vi "Set Multicolumn Listbox Column Width.vi"(5 "Number of Columns":i32, 6 "Auto Columns":bool=TRUE, 7 "Number of Rows":u32=42, 10 "error in (no error)":errorcluster, 11 "Multicolumn ListBox":refnum<vi>) -> (2 "error out":errorcluster, 3 "reference out":refnum<vi>)   [LabVIEW 2017]
uses:
  <vilib>/Utility/miscctls.llb/LVRowAndColumnTypeDef.ctl
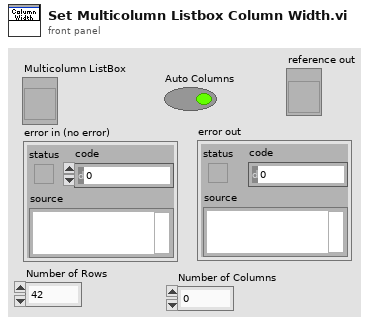
[diagram p1: front panel]
types:
  T1 = typedef "LVRowAndColumnTypeDef.ctl" = cluster{"Row":i32, "Column":i32}
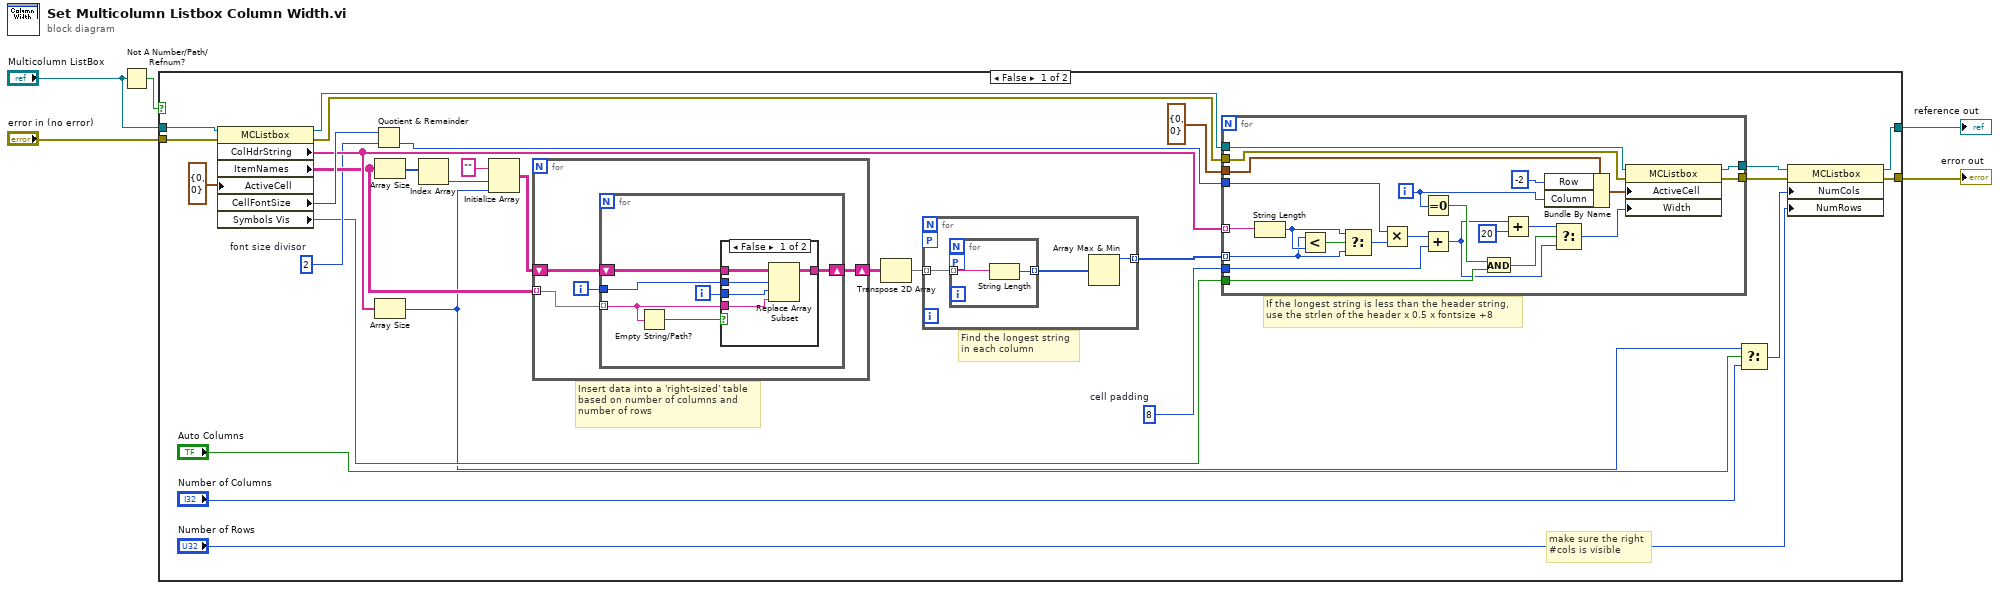
[diagram p0: block diagram]
diagram:
  n1 = Not A Number/Path/Refnum?(number/path/refnum="Multicolumn ListBox") -> (NaN/Path/Refnum?=w3:bool)
  n2 = case shown="False" w3 {
    tunnel: "Multicolumn ListBox" -> [w19 w79]
    tunnel: "error in (no error)" -> [w14 w80]
    tunnel: [w13 w80] -> w4
    tunnel: [w7 w79] -> w1
    frame False {
      w20 = u32 8  # cell padding
      w22 = u32 2  # font size divisor
      # "make sure the right\n#cols is visible"
      # "If the longest string is less than the header string,\nuse the strlen of the header x 0.5 x fontsize +8"
      # "Find the longest string\nin each column"
      # "Insert data into a 'right-sized' table\nbased on number of columns and\nnumber of rows"
      n3 = property on="Property Node" class="MCListbox"(reference=w19, error in=w14, "ActiveCell"=T1 {"Row"=0, "Column"=0} ("Active Cell:Active Cell")) -> (reference out=w15:refnum<vi>, error out=w18:errorcluster, "ColHdrString"=w25:string[], "ItemNames"=w24:string[][], "CellFontSize"=w30:u32, "Symbols Vis"=w12:bool)
      n4 = Quotient & Remainder(x=w30, y=w22) -> (floor(x/y)=w21:u32)  [unwired: 1 out]
      n5 = Array Size(array=w24) -> (size(s)=w28:i32[])
      n6 = Array Size(array=w25) -> (size(s)=w6:i32)
      n7 = Index Array(array=w28) -> (element=w29:i32)  [unwired: 1 in]
      n8 = Initialize Array("", w29, w6) -> (w26:string[][])
      n9 = for {
        shift-right: [w37] -> w23
        shift-left: w26 -> [w38]
        tunnel: w24 -> [w35] mode=indexing
        i -> [w36]
        n10 = for {
          tunnel: w36 -> [w42]
          tunnel: w35 -> [w40] mode=indexing
          shift-right: [w43] -> w37
          shift-left: w38 -> [w44]
          i -> [w41]
          n11 = Empty String/Path?(string/path=w40) -> (empty?=w39:bool)
          n12 = case shown="False" w39 {
            tunnel: w44 -> [w49 w50]
            tunnel: [w48 w50] -> w43
            tunnel: w42 -> [w47 _]
            tunnel: w41 -> [w46 _]
            tunnel: w40 -> [w45 _]
            frame False {
              n13 = Replace Array Subset(array=w49, new element=w45, index (row)=w47, index (col)=w46) -> (w48:string[][])
            }
            frame True {
            }
          }
        }
      }
      n14 = Transpose 2D Array(2D array=w23) -> (transposed array=w33:string[][])
      n15 = for {
        tunnel: w33 -> [w53] mode=indexing
        tunnel: [w51] -> w31 mode=indexing
        workers-P: _ -> [_]
        n16 = for {
          tunnel: w53 -> [w55] mode=indexing
          tunnel: [w54] -> w52 mode=indexing
          workers-P: _ -> [_]
          n17 = String Length(string=w55) -> (length=w54:i32)
        }
        n18 = Array Max & Min(array=w52) -> (max value=w51:i32)  [unwired: 3 out]
      }
      n19 = for {
        tunnel: w25 -> [w73] mode=indexing
        tunnel: T1 {"Row"=0, "Column"=0} ("Active Cell:Active Cell") -> [w78]
        tunnel: w31 -> [w66] mode=indexing
        tunnel: w21 -> [w74]
        tunnel: w20 -> [w72]
        tunnel: w18 -> [w71]
        tunnel: [w70] -> w17
        tunnel: [w69] -> w16
        tunnel: w15 -> [w68]
        tunnel: w12 -> [w61]
        i -> [w63]
        n20 = String Length(string=w73) -> (length=w67:i32)
        n21 = Less?(x=w66, y=w67) -> (x < y?=w65:bool)
        n22 = Select(t=w67, s=w65, f=w66) -> (s? t:f=w64:i32)
        n23 = Multiply(x=w74, y=w64) -> (x*y=w75:u32)
        n24 = Equal To 0?(x=w63) -> (x = 0?=w62:bool)
        n25 = Add(x=w75, y=w72) -> (x+y=w58:u32)
        n26 = And(x=w62, y=w61) -> (x .and. y?=w59:bool)
        n27 = Add(x=w58, y=u32 20) -> (x+y=w57:u32)
        n28 = Bundle By Name(cluster=w78, "Row"=-2, "Column"=w63) -> (w77:T1)
        n29 = Select(t=w57, s=w59, f=w58) -> (s? t:f=w60:u32)
        n30 = property on="Property Node" class="MCListbox"(reference=w68, error in=w71, "ActiveCell"=w77, "Width"=w60) -> (reference out=w69:refnum<vi>, error out=w70:errorcluster)
      }
      n31 = Select(t=w6, s="Auto Columns", f="Number of Columns") -> (s? t:f=w8:i32)
      n32 = property on="Property Node" class="MCListbox"(reference=w16, error in=w17, "NumCols"=w8, "NumRows"="Number of Rows") -> (reference out=w7:refnum<vi>, error out=w13:errorcluster)
    }
    frame True {
    }
  }
  "error out" <- w4
  "reference out" <- w1
